vi "mainMultiColorWorm.vi"() -> ()   [LabVIEW 2017]
uses:
  globalDevices.vi
  globalUtilities.vi
panel:
  in  "Strain name":string
  out "hamamatsuCooling":bool
  in  "molecules":T1(array[cluster])=[{"molecule"="BFP", "exposureTimeMultiplier"=1.0}, {"molecule"="Cerulean", "exposureTimeMultiplier"=1.0}, {"molecule"="GFP", "exposureTimeMultiplier"=1.0}, {"molecule"="mOrange", "exposureTimeMultiplier"=1.0}, {"molecule"="mCherry", "exposureTimeMultiplier"=1.0}, {"molecule"="mNeptune", "exposureTimeMultiplier"=1.0}]
  in  "height of volume (um)":dbl=50.0
  out "folder name":string
  out "current image 5":u16[][](graph)
  out "current image 4":u16[][](graph)
  out "current image 3":u16[][](graph)
  out "current image 2":u16[][](graph)
  out "current image 1":u16[][](graph)
  out "current image 0":u16[][](graph)
  out "current channel":string
  out "current plane":i32
  in  "abort":bool
  in  "number of Z planes":i32=30
  # "MULTICOLOR WORM"
  # "STEPS\n- Optomechanical parts\n    - Blades out\n    - Mirrors labeled \"Multicolor\" in\n    - Photodiode in upper post and turned on\n    - Low-mag objective at right height (see\n       marker on yellow lab tape)\n\n- Turning on devices\n   - Turn on all devices as usual, except the\n      Hamamatsu camera. Do this by pressing\n      the \"General\" button on the \"TrippLite\"\n      switch, and the green button on the stage\n      controller next to it. Turn on the spinning\n      disk unit by turning the key.\n   - If the lasers are not on, turn them on \n     and, after warmup, turn the keys on \"on\".\n   - Restart the filter wheel controller (behind\n      the camera) Prior ProScan II.\n\n- Positioning the worm in XY and roughly in Z\n   - Start basic/piezoHoldMidway. This will \n      bring the piezo of the high-mag objective\n      to its central position.\n   - Using the eyepiece, center the worm in XY\n      using the white joystick and roughly in Z\n      using the manual knob.\n   - Stop piezoHoldMidway.\n\n- Positioning the worm finely in Z\n   - Turn off the light and turn on the \n      Hamamatsu camera and its chiller by \n      pressing the \"Hamamatsu\" button on the\n      \"TrippLite\" switch.\n   - Use basic/multiColorWormSetLaserAndFilter\n      to set the appropriate positions on the \n      slider and filter wheel to be able to see one\n      of the molecules in the worm.\n   - Open HCImageLive at press \"Live\" to start\n      acquiring and displaying the images from\n      the Hamamatsu camera.\n   - Finely center the worm in the z direction\n      using the knob controlling the z position of\n      the high-mag objective.\n   - Press \"Abort\" in HCImageLive and close\n      the program.\n\n- Do the actual multicolor acquisition\n   - Start the multicolor recording starting this\n      program. The first time you start this\n      program after turning on the camera, there\n      will be a delay of 30 seconds to allow the \n      camera sensor to cool down.\n   - If you need to add notes to the logbook,\n      you can open, at any time, main/logbook."
  # "SETTINGS"
  # "The program acquires an image in each channel plane after plane, in the order specified below. If for this specific worm you want to expose a molecule more than in the references, specify a multiplier of the reference exposure time. (For example, if the reference for BFP was acquired with 100 ms exposure and you set the multiplier to 2, the total exposure time will be 200 ms.)"
  # "DIAGNOSTICS"
  # "If you abort, the scan will not be completed\nand the data will not be saved."
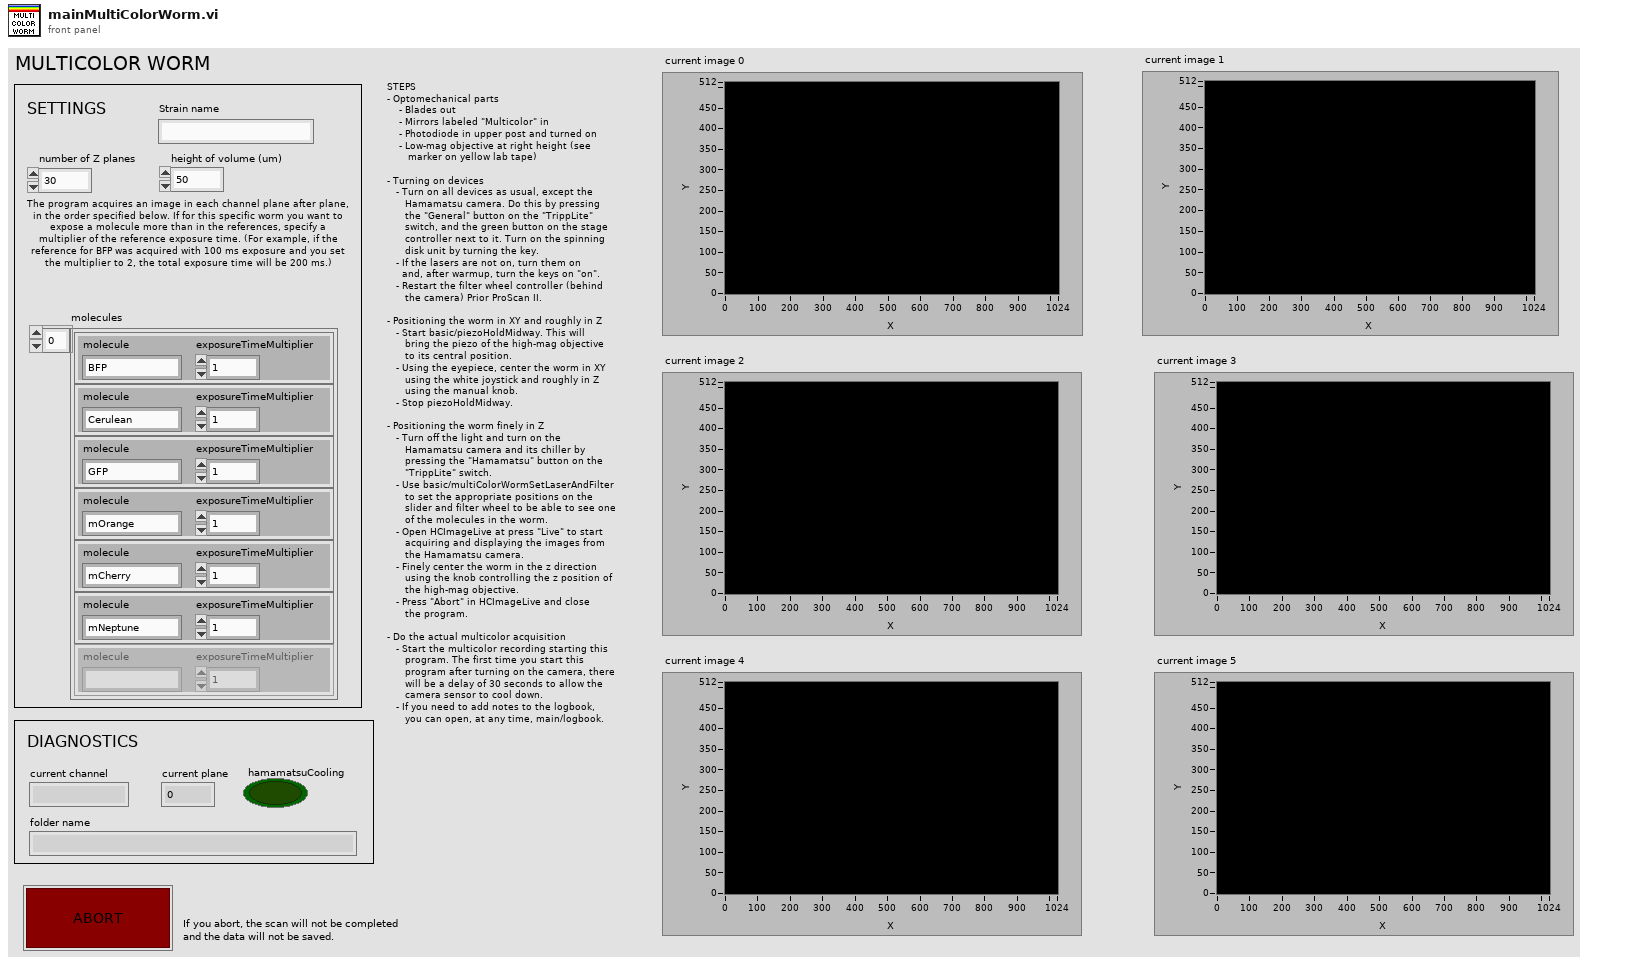
[diagram p1: front panel]
types:
  T1 = cluster{"molecule":string, "exposureTimeMultiplier":dbl}[]
  T2 = cluster{"height":i32, "width":i32, "datatype":i32}
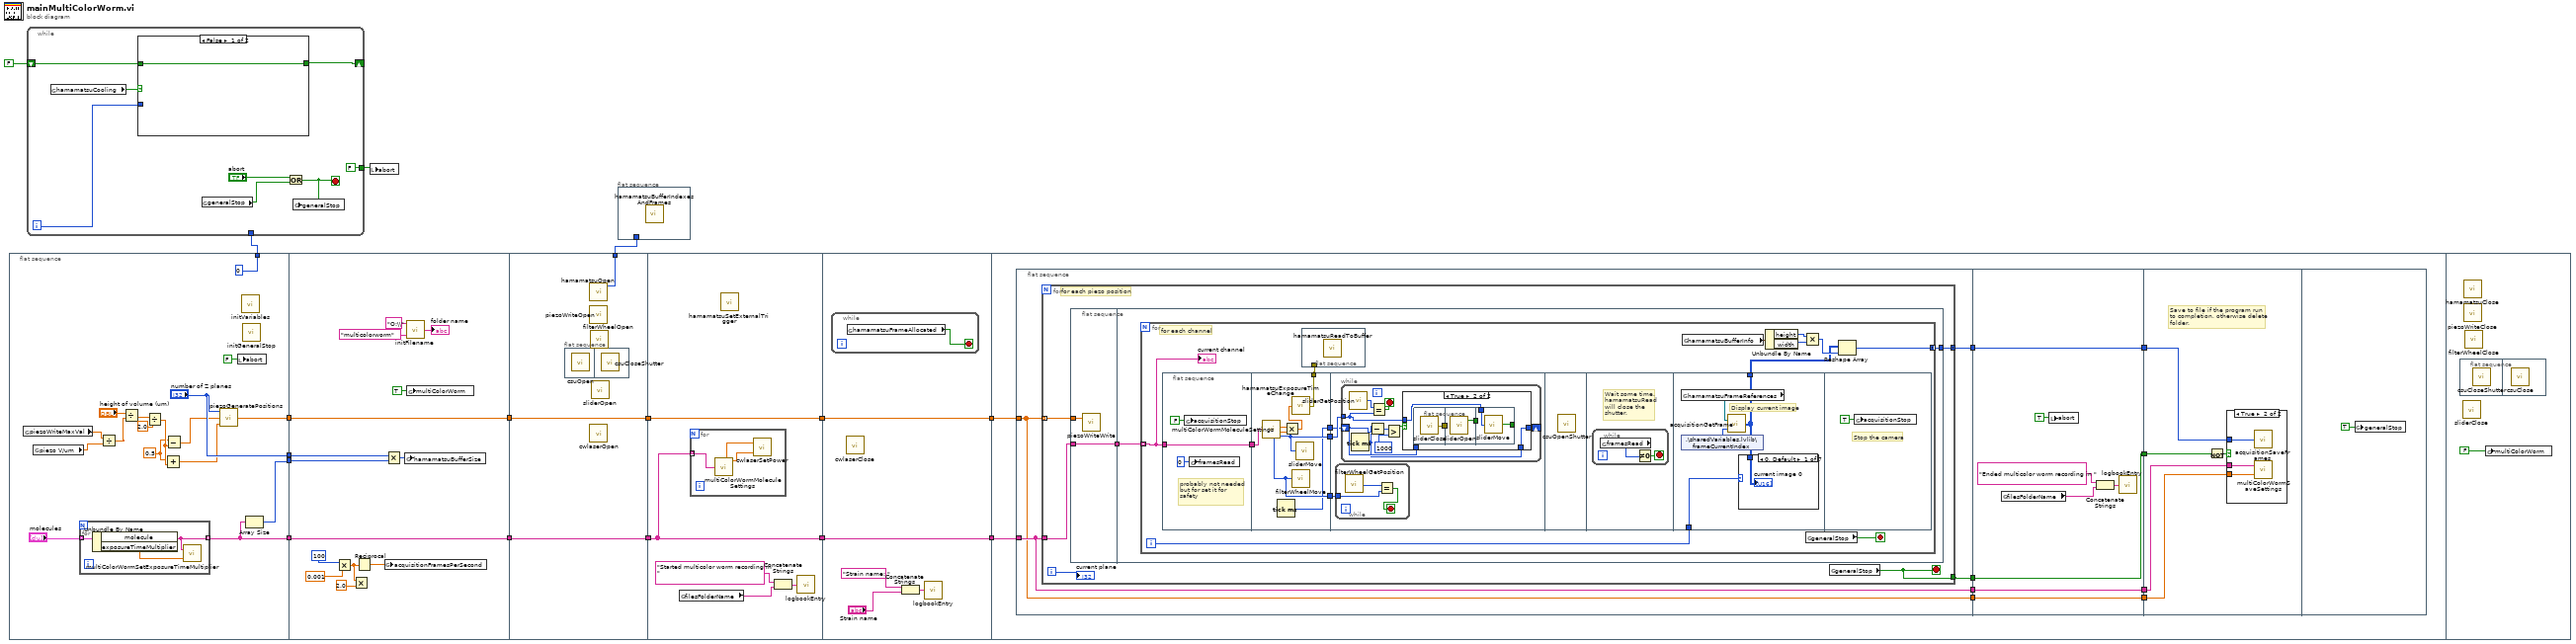
[diagram p0: block diagram]
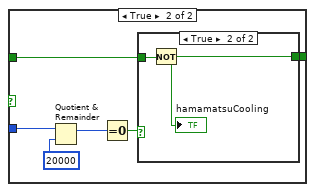
[diagram p2: hidden frame]
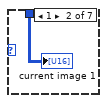
[diagram p5: hidden frame]
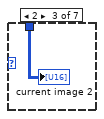
[diagram p6: hidden frame]
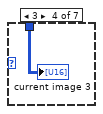
[diagram p7: hidden frame]
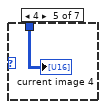
[diagram p8: hidden frame]
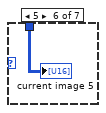
[diagram p9: hidden frame]
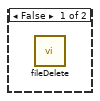
[diagram p11: hidden frame]
diagram:
  n1 = flat-sequence {
    tunnel: [w17] -> w12
    tunnel: [w33] -> w10
    tunnel: ["number of Z planes"] -> w9
    tunnel: [w31] -> w8
    tunnel: [0] -> w3
    tunnel: [w47] -> w13
    tunnel: w12 -> [w47]
    tunnel: [w46] -> w11
    tunnel: w10 -> [w46]
    tunnel: w9 -> [w44]
    tunnel: w8 -> [w43]
    tunnel: [w51] -> w7
    tunnel: [w52] -> w5
    tunnel: [w53] -> w16
    tunnel: w13 -> [w52]
    tunnel: w11 -> [w51]
    tunnel: w7 -> [w58]
    tunnel: [w58] -> w6
    tunnel: w5 -> [w57]
    tunnel: [w57] -> w4
    tunnel: w6 -> [w66]
    tunnel: [w66] -> w15
    tunnel: w4 -> [w65]
    tunnel: [w65] -> w14
    tunnel: w15 -> [w77]
    tunnel: w14 -> [w76]
    frame #0 {
      w19 = 0.5
      n2 = global read "globalDevices.vi" "piezoWriteMaxVal"() -> (w27:dbl)
      n3 = global read "globalDevices.vi" "piezo V/um"() -> (w26:dbl)
      n4 = for {
        tunnel: "molecules" -> [w36] mode=indexing
        tunnel: [w35] -> w17 mode=indexing
        n5 = Unbundle By Name(w36) -> ("molecule"=w35:string, "exposureTimeMultiplier"=w34:dbl)
        n6 = call "multiColorWormSetExposureTimeMultiplier.vi"("exposureTimeMultiplier"=w34, "molecule"=w35) -> ()  [unwired: 1 in]
      }
      n7 = Divide(x=w27, y=w26) -> (x/y=w23:dbl)
      n8 = Divide(x="height of volume (um)", y=w23) -> (x/y=w25:dbl)
      n9 = Divide(x=w25, y=2.0) -> (x/y=w22:dbl)
      n10 = Add(x=w19, y=w22) -> (x+y=w20:dbl)
      n11 = Subtract(x=w19, y=w22) -> (x-y=w21:dbl)
      n12 = call "piezoGeneratePositions.vi"("zf"=w20, "z0"=w21, "M"="number of Z planes") -> ("positions (z)"=w33:dbl[])
      n13 = local write "abort"(FALSE ("abort")) -> ()
      n14 = call "initVariables.vi"() -> ()  [unwired: 12 in]
      n15 = call "initGeneralStop.vi"() -> ()  [unwired: 1 in]
      n16 = Array Size(array=w17) -> (size(s)=w31:i32)
    }
    frame #1 {
      n17 = Multiply(x=u16 100 ("exposure (ms)"), y=0.001) -> (x*y=w39:dbl)
      n18 = Multiply(x=w39, y=2.0) -> ()  [unwired: 1 out]
      n19 = Reciprocal(x=w39) -> (1/x=w48:dbl)
      n20 = global write "globalUtilities.vi" "acquisitionFramesPerSecond"(w48) -> ()
      n21 = Multiply(x=w44, y=w43) -> (x*y=w45:i32)
      n22 = global write "globalDevices.vi" "hamamatsuBufferSize"(w45) -> ()
      n23 = call "initFilename.vi"("Experiment type"="multicolorworm", "Base disk and folder"="O:\\") -> ("folder name"=→"folder name":string)
      n24 = global write "globalUtilities.vi" "multiColorWorm"(TRUE ("multiColorWorm")) -> ()
    }
    frame #2 {
      n25 = flat-sequence {
        frame #0 {
          n26 = call "csuOpen.vi"() -> ()  [unwired: 14 in, 2 out]
        }
        frame #1 {
          n27 = call "csuCloseShutter.vi"() -> ()  [unwired: 16 in]
        }
      }
      n28 = call "hamamatsuOpen.vi"() -> ("Handle out"=w53:u32)  [unwired: 3 out]
      n29 = call "piezoWriteOpen.vi"() -> ()  [unwired: 2 in]
      n30 = call "cwlaserOpen.vi"() -> ()  [unwired: 4 in]
      n31 = call "filterWheelOpen.vi"() -> ()  [unwired: 12 in]
      n32 = call "sliderOpen.vi"() -> ()  [unwired: 1 in, 2 out]
    }
    frame #3 {
      n33 = global read "globalUtilities.vi" "filesFolderName"() -> (w55:string)
      n34 = for {
        tunnel: w57 -> [w61] mode=indexing
        n35 = call "multiColorWormMoleculeSettings.vi"("molecule"=w61) -> ("laserWavelength"=w60:dbl, "laser power (mW)"=w59:dbl)  [unwired: 4 out]
        n36 = call "cwlaserSetPower.vi"("power (mW)"=w59, "wavelength"=w60) -> ()  [unwired: 1 out]
      }
      n37 = call "hamamatsuSetExternalTrigger.vi"() -> ()  [unwired: 12 in]
      n38 = Concatenate Strings("Started multicolor worm recording in ", w55) -> (w56:string)
      n39 = call "logbookEntry.vi"("Log book entry"=w56) -> ()  [unwired: 2 out]
    }
    frame #4 {
      n40 = while {
        stop <- w67 stop-if-true
        n41 = global read "globalDevices.vi" "hamamatsuFrameAllocated"() -> (w67:bool)
      }
      n42 = call "cwlaserClose.vi"() -> ()  [unwired: 3 in]
      n43 = Concatenate Strings("Strain name: " ("string"), "Strain name") -> (w64:string)
      n44 = call "logbookEntry.vi"("Log book entry"=w64) -> ()  [unwired: 2 out]
    }
    frame #5 {
      n45 = flat-sequence {
        tunnel: w77 -> [w79]
        tunnel: w76 -> [w80]
        tunnel: [w81] -> w75
        tunnel: [w80] -> w73
        tunnel: [w79] -> w71
        tunnel: [w78] -> w69
        tunnel: w75 -> [w161]
        tunnel: [w161] -> w74
        tunnel: w73 -> [w160]
        tunnel: [w160] -> w72
        tunnel: w71 -> [w159]
        tunnel: [w159] -> w70
        tunnel: w69 -> [w154]
        tunnel: [w154] -> w68
        tunnel: w74 -> [w166]
        tunnel: w72 -> [w165]
        tunnel: w70 -> [w164]
        tunnel: w68 -> [w162]
        frame #0 {
          n46 = for {
            tunnel: w79 -> [w87] mode=indexing
            tunnel: w80 -> [w86]
            tunnel: [w84] -> w81 mode=concatenating
            tunnel: [w82] -> w78
            i -> [w83]
            stop <- w82 stop-if-true
            # "for each piezo position"
            n47 = flat-sequence {
              tunnel: w87 -> [w89]
              tunnel: w86 -> [w88]
              tunnel: [w88] -> w85
              tunnel: w85 -> [w91]
              tunnel: [w90] -> w84
              frame #0 {
                n48 = call "piezoWriteWrite.vi"("input"=w89) -> ()  [unwired: 2 in]
              }
              frame #1 {
                n49 = for {
                  tunnel: w91 -> [w95] mode=indexing
                  tunnel: [w99] -> w90 mode=concatenating
                  i -> [w94]
                  stop <- w98 stop-if-true
                  # "for each channel"
                  n50 = flat-sequence {
                    tunnel: w95 -> [w108]
                    tunnel: [w108] -> w105
                    tunnel: w105 -> [w116]
                    tunnel: [w112] -> w97
                    tunnel: [w111] -> w96
                    tunnel: [w110] -> w93
                    tunnel: [w109] -> w92
                    tunnel: w96 -> [w119]
                    tunnel: w93 -> [w118]
                    tunnel: w92 -> [w117]
                    tunnel: [w144] -> w100
                    tunnel: w94 -> [w145]
                    frame #0 {
                      # "probably not needed\nbut for set it for \nsafety"
                      n51 = global write "globalUtilities.vi" "acquisitionStop"(FALSE ("acquisitionStop")) -> ()
                      n52 = global write "globalUtilities.vi" "framesRead"(u32 0 ("framesRead")) -> ()
                    }
                    frame #1 {
                      n53 = call "multiColorWormMoleculeSettings.vi"("molecule"=w116) -> ("filter wheel position"=w110:u8, "exposure time (s)"=w114:dbl, "exposureTimeMultiplier"=w115:dbl, "slider position"=w111:u16)  [unwired: 2 out]
                      n54 = Tick Count (ms)() -> (millisecond timer value=w109:u32)
                      n55 = Multiply(x=w114, y=w115) -> (x*y=w113:dbl)
                      n56 = call "hamamatsuExposureTimeChange.vi"("Exposure time (s)"=w113) -> ("error out"=w112:errorcluster)
                      n57 = call "filterWheelMove.vi"("filter index"=w110) -> ()  [unwired: 1 out]
                      n58 = call "sliderMove.vi"("position"=w111) -> ()  [unwired: 1 out]
                    }
                    frame #2 {
                      n59 = while {
                        tunnel: w118 -> [w121]
                        stop <- w120 stop-if-true
                        n60 = call "filterWheelGetPosition.vi"() -> ("number"=w122:i32)  [unwired: 1 in]
                        n61 = Equal?(x=w122, y=w121) -> (x = y?=w120:bool)
                      }
                      n62 = while {
                        tunnel: w119 -> [w127]
                        shift-right: [w124] -> _
                        shift-left: w117 -> [w125]
                        stop <- w126 stop-if-true
                        n63 = call "sliderGetPosition.vi"() -> ("position"=w131:i32)  [unwired: 1 in]
                        n64 = Tick Count (ms)() -> (millisecond timer value=w123:u32)
                        n65 = Subtract(x=w123, y=w125) -> (x-y=w130:u32)
                        n66 = Equal?(x=w131, y=w127) -> (x = y?=w126:bool)
                        n67 = Greater?(x=w130, y=u32 1000) -> (0:w128:bool)
                        n68 = case shown="True" w128 {
                          tunnel: w127 -> [_ w136]
                          tunnel: w125 -> [w132 _]
                          tunnel: [w132 w135] -> w124
                          tunnel: w123 -> [_ w135]
                          frame False {
                          }
                          frame True {
                            n69 = flat-sequence {
                              tunnel: [w137] -> w134
                              tunnel: w134 -> [_]
                              tunnel: [w138] -> w133
                              tunnel: w136 -> [w140]
                              tunnel: [w139] -> _
                              tunnel: w133 -> [_]
                              frame #0 {
                                n70 = call "sliderClose.vi"() -> ("error out"=w137:errorcluster)  [unwired: 2 in]
                              }
                              frame #1 {
                                n71 = call "sliderOpen.vi"() -> ("success"=w138:bool)  [unwired: 1 in, 1 out]
                              }
                              frame #2 {
                                n72 = call "sliderMove.vi"("position"=w140) -> ("success"=w139:bool)
                              }
                            }
                          }
                        }
                      }
                    }
                    frame #3 {
                      n73 = call "csuOpenShutter.vi"() -> ()  [unwired: 16 in]
                    }
                    frame #4 {
                      # "Wait some time.\nhamamatsuRead\nwill close the\nshutter."
                      n74 = while {
                        stop <- w141 stop-if-true
                        n75 = global read "globalUtilities.vi" "framesRead"() -> (w142:u32)
                        n76 = Not Equal To 0?(x=w142) -> (x != 0?=w141:bool)
                      }
                    }
                    frame #5 {
                      # "Display current image"
                      n77 = shared-variable ".\\sharedVariables.lvlib\\frameCurrentIndex"() -> (w143:i32)  [unwired: 1 in, 1 out]
                      n78 = global read "globalDevices.vi" "hamamatsuFrameReferences"() -> (w146:refnum<data-value>[])
                      n79 = call "acquisitionGetFrame.vi"("index"=w143, "hamamatsuFrameReferences"=w146) -> ("frameOut"=w144:u16[][])
                      n80 = case shown="0, Default" w145 {
                        tunnel: w144 -> [w147 w148 w149 w150 w151 w152 _]
                        frame 0, Default {
                          "current image 0" <- w147
                        }
                        frame 1 {
                          "current image 1" <- w148
                        }
                        frame 2 {
                          "current image 2" <- w149
                        }
                        frame 3 {
                          "current image 3" <- w150
                        }
                        frame 4 {
                          "current image 4" <- w151
                        }
                        frame 5 {
                          "current image 5" <- w152
                        }
                        frame 6 {
                        }
                      }
                    }
                    frame #6 {
                      # "Stop the camera"
                      n81 = global write "globalUtilities.vi" "acquisitionStop"(TRUE ("acquisitionStop")) -> ()
                    }
                  }
                  n82 = flat-sequence {
                    tunnel: w97 -> [_]
                    frame #0 {
                      n83 = call "hamamatsuReadToBuffer.vi"() -> ()  [unwired: 12 in]
                    }
                  }
                  n84 = global read "globalDevices.vi" "hamamatsuBufferInfo"() -> (w104:T2)
                  n85 = Unbundle By Name(w104) -> ("height"=w103:i32, "width"=w102:i32)
                  n86 = Multiply(x=w103, y=w102) -> (x*y=w101:i32)
                  n87 = global read "globalUtilities.vi" "generalStop"() -> (w98:bool)
                  n88 = Reshape Array(w100, w101) -> (w99:u16[])
                  "current channel" <- w95
                }
              }
            }
            n89 = global read "globalUtilities.vi" "generalStop"() -> (w82:bool)
            "current plane" <- w83
          }
        }
        frame #1 {
          n90 = global read "globalUtilities.vi" "filesFolderName"() -> (w158:string)
          n91 = local write "abort"(TRUE ("abort")) -> ()
          n92 = Concatenate Strings("Ended multicolor worm recording in ", w158) -> (w157:string)
          n93 = call "logbookEntry.vi"("Log book entry"=w157) -> ()  [unwired: 2 out]
        }
        frame #2 {
          # "Save to file if the program run\nto completion, otherwise delete\nfolder."
          n94 = Not(x=w162) -> (.not. x?=w163:bool)
          n95 = case shown="True" w163 {
            tunnel: w166 -> [_ w169]
            tunnel: w165 -> [_ w168]
            tunnel: w164 -> [_ w167]
            frame False {
              n96 = call "fileDelete.vi"() -> ()  [unwired: 12 in]
            }
            frame True {
              n97 = call "acquisitionSaveFrames.vi"("frames (1D)"=w169) -> ()  [unwired: 1 in]
              n98 = call "multiColorWormSaveSettings.vi"("piezoPosition"=w167, "moleculesSequence"=w168) -> ()  [unwired: 1 in]
            }
          }
        }
        frame #3 {
          n99 = global write "globalUtilities.vi" "generalStop"(TRUE ("generalStop")) -> ()
        }
      }
    }
    frame #6 {
      n100 = flat-sequence {
        frame #0 {
          n101 = call "csuCloseShutter.vi"() -> ()  [unwired: 16 in]
        }
        frame #1 {
          n102 = call "csuClose.vi"() -> ()  [unwired: 12 in]
        }
      }
      n103 = call "sliderClose.vi"() -> ()  [unwired: 2 in, 1 out]
      n104 = call "hamamatsuClose.vi"() -> ()  [unwired: 1 out]
      n105 = call "piezoWriteClose.vi"() -> ()  [unwired: 1 in]
      n106 = call "filterWheelClose.vi"() -> ()  [unwired: 12 in]
      n107 = global write "globalUtilities.vi" "multiColorWorm"(FALSE ("multiColorWorm")) -> ()
    }
  }
  n108 = while {
    tunnel: w3 -> [_]
    tunnel: [FALSE] -> w2
    shift-right: [w172] -> _
    shift-left: FALSE -> [w173]
    i -> [w174]
    stop <- w178 stop-if-true
    n109 = global read "globalDevices.vi" "hamamatsuCooling"() -> (w175:bool)
    n110 = case shown="False" w175 {
      tunnel: w174 -> [_ w186]
      tunnel: w173 -> [w180 w182]
      tunnel: [w180 w181] -> w172
      frame False {
      }
      frame True {
        n111 = Quotient & Remainder(x=w186, y=20000) -> (x-y*floor(x/y)=w184:i32)  [unwired: 1 out]
        n112 = Equal To 0?(x=w184) -> (x = 0?=w183:bool)
        n113 = case shown="True" w183 {
          tunnel: w182 -> [w187 w189]
          tunnel: [w187 w188] -> w181
          frame False {
          }
          frame True {
            n114 = Not(x=w189) -> (.not. x?=w188:bool)
            "hamamatsuCooling" <- w188
          }
        }
      }
    }
    n115 = global read "globalUtilities.vi" "generalStop"() -> (w177:bool)
    n116 = Or(x="abort", y=w177) -> (x .or. y?=w178:bool)
    n117 = global write "globalUtilities.vi" "generalStop"(w178) -> ()
  }
  n118 = local write "abort"(w2) -> ()
  n119 = flat-sequence {
    tunnel: w16 -> [_]
    frame #0 {
      n120 = call "hamamatsuBufferIndexesAndFrames.vi"() -> ()  [unwired: 12 in]
    }
  }
